vi "Stop DAQ Timeout.vi"(8 "error in (no error)":errorcluster, 10 "Timeout":i32, 11 "Cfg Grandmaster in":refnum<class "Cfg Grandmaster.lvclass">) -> (0 "error out":errorcluster, 3 "Cfg Grandmaster out":refnum<class "Cfg Grandmaster.lvclass">)   [LabVIEW 2018, in "Configuration Grandmaster.lvlib" / "Cfg Grandmaster.lvclass"]
uses:
  Cfg Grandmaster.lvclass
  Common/Controls/DAQMan Mode.ctl
  Cfg Grandmaster.lvclass/Cfg Grandmaster.ctl
  Class FP Ctrls/FP Controls.lvclass
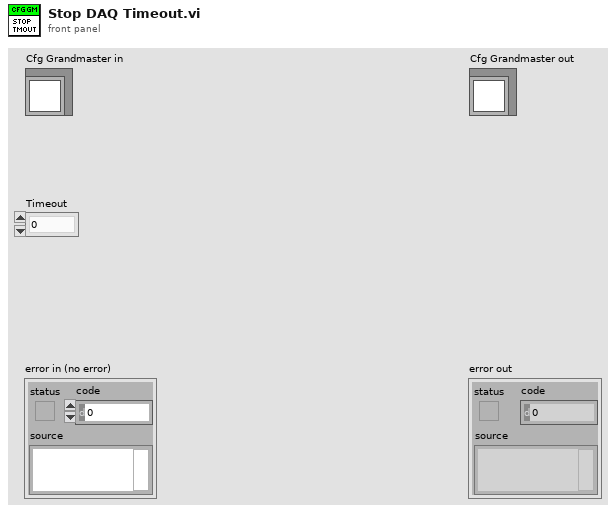
[diagram p1: front panel]
types:
  T1 = typedef "DAQMan Mode.ctl" = enum16{"Cfg", "Run", "Shutting Down"}
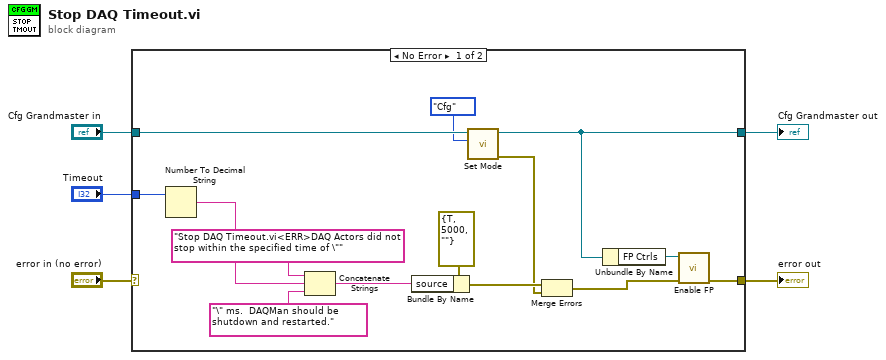
[diagram p0: block diagram]
diagram:
  n1 = case shown="No Error" "error in (no error)" {
    selector: "error in (no error)" -> [_ w21]
    tunnel: [w9 w21] -> w4
    tunnel: [w7 w20] -> w2
    tunnel: "Cfg Grandmaster in" -> [w12 w20]
    tunnel: "Timeout" -> [w17 _]
    frame No Error {
      n2 = Number To Decimal String(number=w17) -> (decimal integer string=w15:string)  [unwired: 1 in]
      n3 = Concatenate Strings("Stop DAQ Timeout.vi<ERR>DAQ Actors did not stop within the specified time of \"" ("source"), w15, "\" ms.  DAQMan should be shutdown and restarted." ("source")) -> (w16:string)
      n4 = Bundle By Name(cluster=errorcluster {"status"=TRUE, "code"=5000, "source"=""} ("error IO"), "source"=w16) -> (w18:errorcluster)
      n5 = call "Set Mode.vi"("Mode"=DAQMan_Mode."Cfg", "Cfg Grandmaster in"=w12) -> ("error out"=w11:errorcluster, "Cfg Grandmaster out"=w7:refnum<class "Cfg Grandmaster.lvclass">)  [unwired: 8 in]
      n6 = Merge Errors(w18, w11) -> (w8:errorcluster)
      n7 = Unbundle By Name(w7) -> ("FP Ctrls"=w6:refnum<class "FP Controls.lvclass">)
      n8 = call "Enable FP.vi"("error in (no error)"=w8, "FP Controls in"=w6) -> ("error out"=w9:errorcluster)  [unwired: 8 in, 1 out]
    }
    frame Error {
    }
  }
  "error out" <- w4
  "Cfg Grandmaster out" <- w2
